vi "Test Reverse String.vi"(8 "error in (no error)":errorcluster) -> (0 "error out":errorcluster, 3 "Pass?":bool)   [LabVIEW 2020]
uses:
  G-Unicode/Types/UTF-8 String/UTF-8 String.lvclass/UTF-8 String.ctl
  8690b08d-f36c-4ee5-acde-790fa2950b16.vi
  ba5b6683-6b7f-4241-8972-fb5dd34213e6.vi
  504d7c14-23e1-4c14-92bf-7573e680de72.vi
  422f9b4b-c10b-46b7-b73f-1268a1c43e11.vi
  239b2762-dc91-42b6-b8b8-d649fddcbd19.vi
  G-Unicode/Private/Conversion/String as Encoded String.vi
  G-Unicode/Private/Conversion/Polymorphic VIs/String as Encoded String (LabVIEW String).vi
  G-Unicode/Private/Library/gu_reverse_string.vi
  ba5b6683-6b7f-4241-8972-fb5dd34213e6.vi/3a31b270-3bb6-4c58-a256-c5fcc2c98f09.vi
  ba5b6683-6b7f-4241-8972-fb5dd34213e6.vi/0ec5df2d-ef9b-4f84-a6a8-ffcedd45c4dc.vi
  G-Unicode/Private/Conversion/Polymorphic VIs/String as Encoded String (UTF-8 String).vi
  239b2762-dc91-42b6-b8b8-d649fddcbd19.vi/3a31b270-3bb6-4c58-a256-c5fcc2c98f09.vi
  239b2762-dc91-42b6-b8b8-d649fddcbd19.vi/0ec5df2d-ef9b-4f84-a6a8-ffcedd45c4dc.vi
  G-Unicode/Private/Conversion/Text to UTF-8.vi
  G-Unicode/Private/Conversion/Polymorphic VIs/Text to UTF-8 (LabVIEW String).vi
  G-Unicode/Private/Library/Result To Error.vi
  G-Unicode/Private/Conversion/Text as Encoded String.vi
  G-Unicode/Private/Conversion/Polymorphic VIs/Text as Encoded String (LabVIEW String).vi
  G-Unicode/Private/Conversion/Polymorphic VIs/Text as Encoded String (UTF-8 String).vi
  G-Unicode/Types/UTF-8 String/Read Encoded UTF-8 String.vi
  <vilib>/Utility/error.llb/Error Cluster From Error Code.vi
  G-Unicode/Types/UTF-8 String/UTF-8 String.lvclass
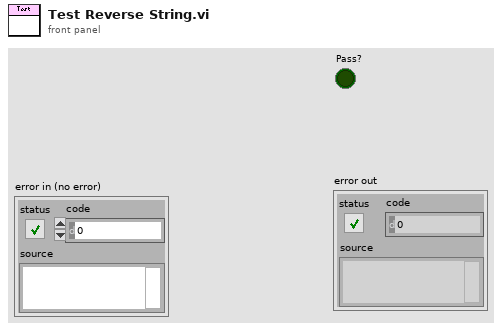
[diagram p1: front panel]
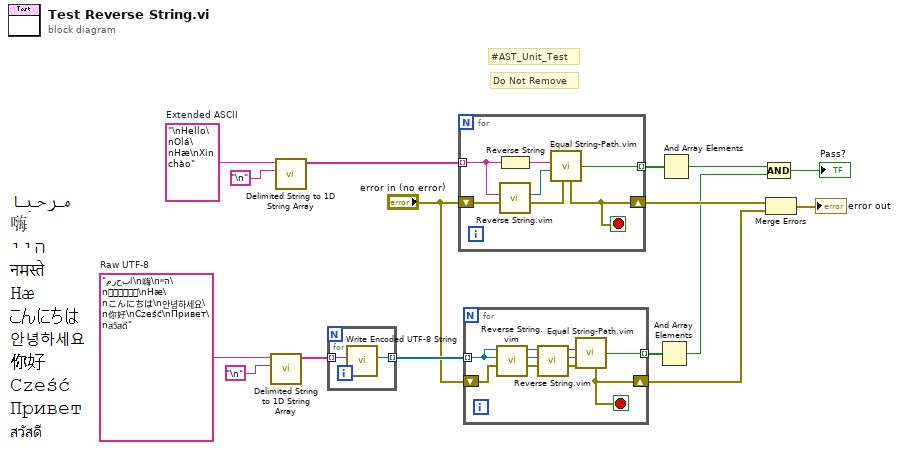
[diagram p0: block diagram]
diagram:
  w2 = "\nHello\nOlá\nHæ\nXin chào"  # Extended ASCII
  w15 = "مرحبا\n嗨\nהיי\nनमस्ते\nHæ\nこんにちは\n안녕하세요\n你好\nCześć\nПривет\nสวัสดี"  # Raw UTF-8
  # "Do Not Remove"
  # "#AST_Unit_Test"
  n1 = call <vilib>:"Delimited String to 1D String Array.vi"("delimiter"="\n", "delimited string"=w15) -> ("string array"=w14:string[])  [unwired: 9 in]
  n2 = call <vilib>:"Delimited String to 1D String Array.vi"("delimiter"="\n", "delimited string"=w2) -> ("string array"=w1:string[])  [unwired: 9 in]
  n3 = for {
    tunnel: w14 -> [w18] mode=indexing
    tunnel: [w17] -> w5 mode=indexing
    n4 = call "Write Encoded UTF-8 String.vi"("Encoded UTF-8 String"=w18) -> ("UTF-8 String"=w17:refnum<class "UTF-8 String.lvclass">)  [unwired: 10 in]
  }
  n5 = for {
    tunnel: [w25] -> w10 mode=indexing
    shift-right: [w19] -> w13
    shift-left: "error in (no error)" -> [w22]
    tunnel: w1 -> [w23] mode=indexing
    stop <- w19 stop-if-true
    n6 = Reverse String(1:w23) -> (0:w24:string)
    n7 = call "Reverse String.vim"("error in"=w22, "String"=w23) -> ("error out"=w20:errorcluster, "Reversed"=w21:refnum<class "UTF-8 String.lvclass">)  [unwired: 8 in]
    n8 = call "Equal String-Path.vim"("error in"=w20, "y"=w21, "x"=w24) -> ("error out"=w19:errorcluster, "Equal?"=w25:bool)  [unwired: 6 in]
  }
  n9 = for {
    tunnel: w5 -> [w30] mode=indexing
    tunnel: [w33] -> w8 mode=indexing
    shift-right: [w26] -> w6
    shift-left: "error in (no error)" -> [w29]
    stop <- w26 stop-if-true
    n10 = call "Reverse String.vim"("error in"=w29, "String"=w30) -> ("error out"=w28:errorcluster, "Reversed"=w32:refnum<class "UTF-8 String.lvclass">)  [unwired: 8 in]
    n11 = call "Reverse String.vim"("error in"=w28, "String"=w32) -> ("error out"=w27:errorcluster, "Reversed"=w31:refnum<class "UTF-8 String.lvclass">)  [unwired: 8 in]
    n12 = call "Equal String-Path.vim"("error in"=w27, "y"=w31, "x"=w30) -> ("error out"=w26:errorcluster, "Equal?"=w33:bool)  [unwired: 6 in]
  }
  n13 = And Array Elements(Boolean array=w8) -> (logical AND=w7:bool)
  n14 = And Array Elements(Boolean array=w10) -> (logical AND=w9:bool)
  n15 = Merge Errors(w13, w6) -> (→"error out":errorcluster)
  n16 = Compound Arithmetic op=AND(w9, w7) -> (→"Pass?":bool)
